vi "AB_API Factory.vi"(8 "error in (no error)":errorcluster, 11 "Build object selector":T2) -> (0 "error out":errorcluster, 1 "Build object type":T1, 2 "Build":refnum<class "AB_Build.lvclass">, 3 "API":refnum<class "NI_AB_API_Build.lvclass">)   [LabVIEW 2020]
uses:
  <vilib>/AppBuilder/AB_API/common/AB_API Build Object Type.ctl
  <vilib>/AppBuilder/AB_Classes/Build/AB_Build.lvclass
  <vilib>/AppBuilder/AB_API/Build/NI_AB_API_Build.lvclass
  <vilib>/AppBuilder/AB_API/common/AB_API Build Object Selector.ctl
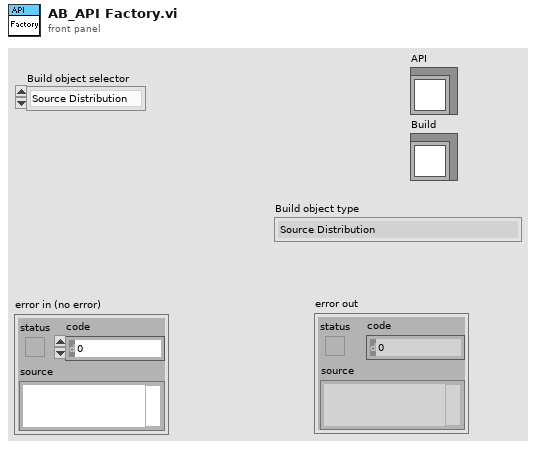
[diagram p1: front panel]
types:
  T1 = typedef "AB_API Build Object Type.ctl" = enum16{"Source Distribution", "DLL", "EXE", "Installer", "Zip File", "RESTful WS", "RTEXE", "Packed Library", "C Generation ", ".NET Interop Assembly"}
  T2 = typedef "AB_API Build Object Selector.ctl" = enum16{"Source Distribution", "Deployable Source Distribution", "DLL", "EXE", "Packed Library", "Deployable Packed Library", "RT EXE", ".NET Interop Assembly"}
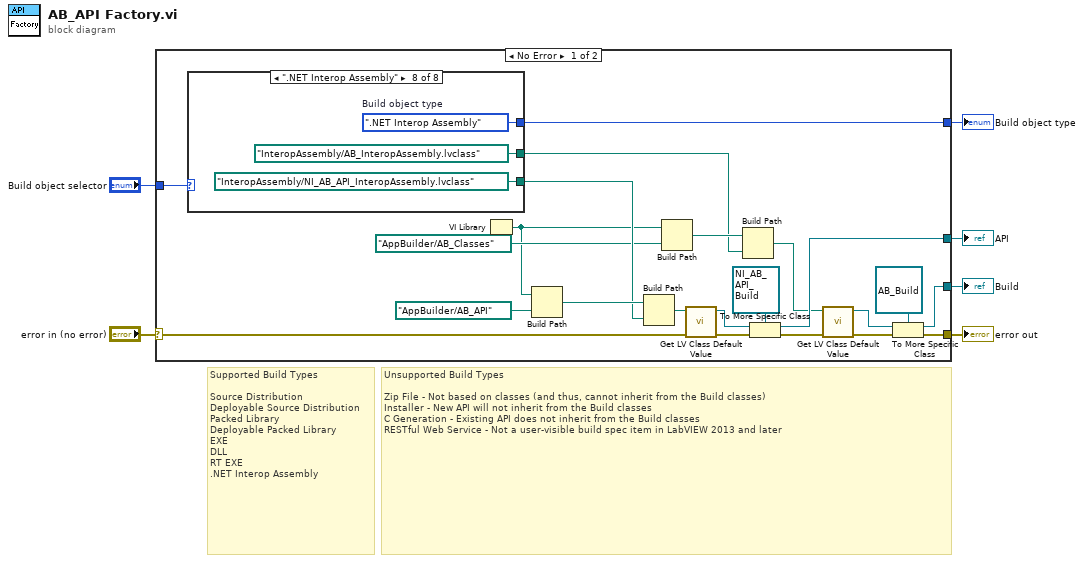
[diagram p0: block diagram]
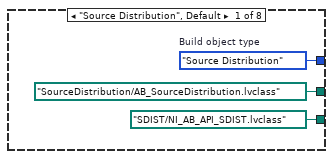
[diagram p2: hidden frame]
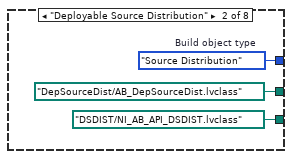
[diagram p3: hidden frame]
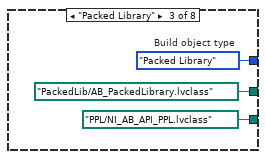
[diagram p4: hidden frame]
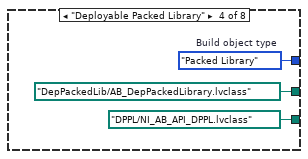
[diagram p5: hidden frame]
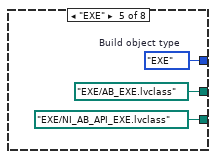
[diagram p6: hidden frame]
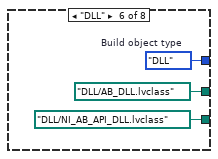
[diagram p7: hidden frame]
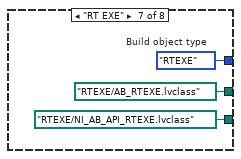
[diagram p8: hidden frame]
diagram:
  # "Unsupported Build Types\n\nZip File - Not based on classes (and thus, cannot inherit from the Build classes)\nInstaller - New API will not inherit from the Build classes\nC Generation - Existing API does not inherit from the Build classes\nRESTful Web Service - Not a user-visible build spec item in LabVIEW 2013 and later"
  # "Supported Build Types\n\nSource Distribution\nDeployable Source Distribution\nPacked Library\nDeployable Packed Library\nEXE\nDLL\nRT EXE\n.NET Interop Assembly"
  n1 = case shown="No Error" "error in (no error)" {
    selector: "error in (no error)" -> [w12 w53]
    tunnel: "Build object selector" -> [w28 _]
    tunnel: [w27 _] -> w5
    tunnel: [w23 _] -> w4
    tunnel: [w19 _] -> w3
    tunnel: [w13 w53] -> w2
    frame No Error {
      n2 = case shown="\".NET Interop Assembly\"" w28 {
        tunnel: [w31 w34 w37 w40 w43 w46 w49 w52] -> w27
        tunnel: [path "SDIST/NI_AB_API_SDIST.lvclass" path "DSDIST/NI_AB_API_DSDIST.lvclass" path "PPL/NI_AB_API_PPL.lvclass" path "DPPL/NI_AB_API_DPPL.lvclass" path "EXE/NI_AB_API_EXE.lvclass" path "DLL/NI_AB_API_DLL.lvclass" path "RTEXE/NI_AB_API_RTEXE.lvclass" path "InteropAssembly/NI_AB_API_InteropAssembly.lvclass"] -> w16
        tunnel: [path "SourceDistribution/AB_SourceDistribution.lvclass" path "DepSourceDist/AB_DepSourceDist.lvclass" path "PackedLib/AB_PackedLibrary.lvclass" path "DepPackedLib/AB_DepPackedLibrary.lvclass" path "EXE/AB_EXE.lvclass" path "DLL/AB_DLL.lvclass" path "RTEXE/AB_RTEXE.lvclass" path "InteropAssembly/AB_InteropAssembly.lvclass"] -> w8
        frame "Source Distribution", Default {
          w31 = AB_API_Build_Object_Type."Source Distribution"  # Build object type
        }
        frame "Deployable Source Distribution" {
          w34 = AB_API_Build_Object_Type."Source Distribution"  # Build object type
        }
        frame "Packed Library" {
          w37 = AB_API_Build_Object_Type."Packed Library"  # Build object type
        }
        frame "Deployable Packed Library" {
          w40 = AB_API_Build_Object_Type."Packed Library"  # Build object type
        }
        frame "EXE" {
          w43 = AB_API_Build_Object_Type."EXE"  # Build object type
        }
        frame "DLL" {
          w46 = AB_API_Build_Object_Type."DLL"  # Build object type
        }
        frame "RT EXE" {
          w49 = AB_API_Build_Object_Type."RTEXE"  # Build object type
        }
        frame ".NET Interop Assembly" {
          w52 = AB_API_Build_Object_Type.".NET Interop Assembly"  # Build object type
        }
      }
      n3 = VI Library() -> (path=w7:path)
      n4 = Build Path(base path=w7, name or relative path=path "AppBuilder/AB_API") -> (appended path=w17:path)
      n5 = Build Path(base path=w17, name or relative path=w16) -> (appended path=w15:path)
      n6 = Build Path(base path=w7, name or relative path=path "AppBuilder/AB_Classes") -> (appended path=w10:path)
      n7 = call <vilib>:"Get LV Class Default Value.vi"("error in (no error)"=w12, "class path"=w15) -> ("error out"=w22:errorcluster, "object"=w21:refnum<class>)  [unwired: 8 in]
      n8 = Build Path(base path=w10, name or relative path=w8) -> (appended path=w9:path)
      n9 = To More Specific Class(target class=refnum<class "NI_AB_API_Build.lvclass"> refnum ("API"), reference=w21, error in=w22) -> (specific class reference=w19:refnum<class "NI_AB_API_Build.lvclass">, error out=w14:errorcluster)
      n10 = call <vilib>:"Get LV Class Default Value.vi"("error in (no error)"=w14, "class path"=w9) -> ("error out"=w25:errorcluster, "object"=w24:refnum<class>)  [unwired: 8 in]
      n11 = To More Specific Class(target class=refnum<class "AB_Build.lvclass"> refnum ("AB_Build out"), reference=w24, error in=w25) -> (specific class reference=w23:refnum<class "AB_Build.lvclass">, error out=w13:errorcluster)
    }
    frame Error {
    }
  }
  "API" <- w3
  "Build" <- w4
  "error out" <- w2
  "Build object type" <- w5
